vi "Agilent DMM Set Resolution.vi"(7 "Measurement Type":T3, 8 "error in (no error)":errorcluster, 9 "Range":T1, 10 "Resolution":T2, 11 "VISA Resource Name":refnum<visa-resource-name>) -> (0 "error out":errorcluster, 3 "dup VISA Resource Name":refnum<visa-resource-name>)   [LabVIEW 2011]
doc: "This VI for the HP 8753 is used to read the sweep type.\n\n0 LINEAR FREQ\n1 LOG FREQ\n2 LIST FREQ\n3 CW TIME\n4 POWER SWEEP"
uses:
  TypeDefs/Agilent DMM Measurement Type.ctl
  TypeDefs/Agilent DMM Resolution.ctl
  TypeDefs/Agilent DMM Range.ctl
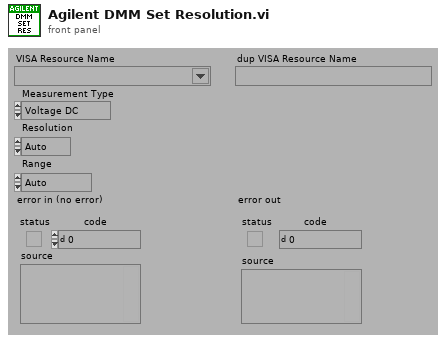
[diagram p1: front panel]
types:
  T1 = typedef "Agilent DMM Range.ctl" = enum16{"Auto", "Min", "Max", "0.01", "0.1", "1", "3", "10", "100", "1,000", "10,000", "100,000", "1,000,000", "10,000,000", "100,000,000"}
  T2 = typedef "Agilent DMM Resolution.ctl" = enum16{"Auto", "Min", "Max", "4 1/2", "5 1/2", "6 1/2"}
  T3 = typedef "Agilent DMM Measurement Type.ctl" = enum16{"Voltage DC", "Voltage DC Ratio", "Voltage AC", "Current DC", "Current AC", "Resistance", "Fresistance", "Frequency", "Period", "Continuity", "Diode"}
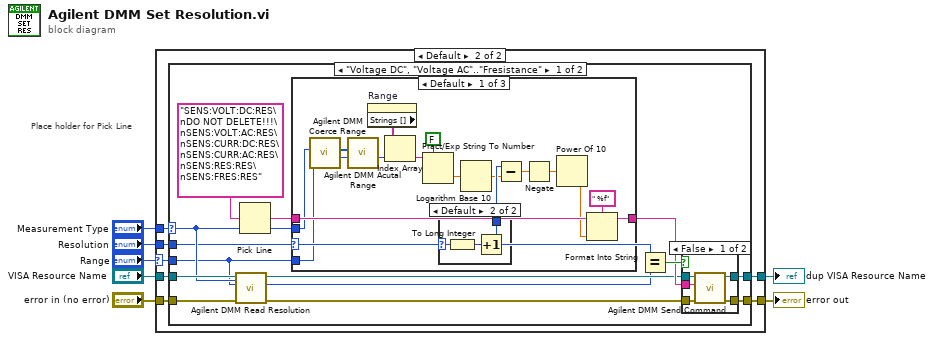
[diagram p0: block diagram]
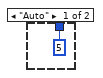
[diagram p4: hidden frame]
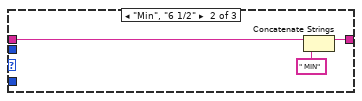
[diagram p5: hidden frame]
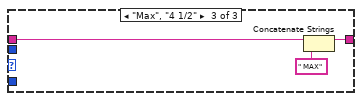
[diagram p6: hidden frame]
diagram:
  # "Place holder for Pick Line"
  n1 = case shown="Default" "Range" {
    selector: "Range" -> [_ w10]
    tunnel: "error in (no error)" -> [w8 w16]
    tunnel: [w8 w15] -> w6
    tunnel: "VISA Resource Name" -> [w9 w14]
    tunnel: [w9 w13] -> w4
    tunnel: "Measurement Type" -> [_ w12]
    tunnel: "Resolution" -> [_ w11]
    frame "Auto" {
      # "The Resolution can only be set\nif the Range is set to something\nbesides Auto."
    }
    frame Default {
      n2 = case shown="\"Voltage DC\", \"Voltage AC\"..\"Fresistance\"" w12 {
        selector: w12 -> [w20 _]
        tunnel: w16 -> [w23 w67]
        tunnel: [w26 w67] -> w15
        tunnel: w14 -> [w24 w66]
        tunnel: [w27 w66] -> w13
        tunnel: w11 -> [w17 _]
        tunnel: w10 -> [w19 _]
        frame "Voltage DC", "Voltage AC".."Fresistance" {
          n3 = call "Agilent DMM Read Resolution.vi"("Measurement Type"=w20, "error in (no error)"=w23, "Range"=w19, "VISA Resource Name"=w24) -> ("error out"=w22:errorcluster, "Resolution"=w18:T2, "dup VISA Resource Name"=w21:refnum<visa-resource-name>)  [unwired: 5 out]
          n4 = Pick Line(multi-line string="SENS:VOLT:DC:RES\nDO NOT DELETE!!!\nSENS:VOLT:AC:RES\nSENS:CURR:DC:RES\nSENS:CURR:AC:RES\nSENS:RES:RES\nSENS:FRES:RES" ("write buffer"), line index=w20) -> (output string=w29:string)  [unwired: 1 out]
          n5 = case shown="Default" w17 {
            selector: w17 -> [w41 _ _]
            tunnel: w29 -> [w54 w61 w64]
            tunnel: [w53 w60 w63] -> w25
            tunnel: w19 -> [w48 _ _]
            tunnel: w20 -> [w47 _ _]
            frame Default {
              n6 = call "Agilent DMM Coerce Range.vi"("Range"=w48, "Measurement Type"=w47) -> ("Coerced Range"=w40:T1, "Available Ranges"=w39:T1[])  [unwired: 8 out]
              n7 = call "Agilent DMM Acutal Range.vi"("Coerced Range"=w40, "Available Ranges"=w39) -> ("Acutal Range"=w38:T1)  [unwired: 9 out]
              n8 = property on="Range" class="Enum (strict)"() -> ("Strings []"=w49:string[])  [unwired: 2 in, 2 out]
              n9 = Index Array(array=w49, index=w38) -> (element=w50:string)
              n10 = Fract/Exp String To Number(use system decimal point (T)=FALSE, string=w50) -> (number=w52:dbl)  [unwired: 3 out]
              n11 = case shown="Default" w41 {
                selector: w41 -> [_ w57]
                tunnel: [5 w59] -> w46
                frame "Auto" {
                }
                frame Default {
                  n12 = To Long Integer(number=w57) -> (32bit integer=w58:i32)
                  n13 = Increment(x=w58) -> (x+1=w59:i32)
                }
              }
              n14 = Logarithm Base 10(1:w52) -> (0:w45:dbl)
              n15 = Subtract(x=w46, y=w45) -> (x-y=w44:dbl)
              n16 = Negate(x=w44) -> (-x=w42:dbl)
              n17 = Power Of 10(x=w42) -> (10^x=w43:dbl)
              n18 = Format Into String(format string=" %f", initial string=w54, w43) -> (resulting string=w53:string)  [unwired: 1 in, 1 out]
            }
            frame "Min", "6 1/2" {
              n19 = Concatenate Strings(w61, " MIN" ("string")) -> (w60:string)
            }
            frame "Max", "4 1/2" {
              n20 = Concatenate Strings(w64, " MAX" ("string")) -> (w63:string)
            }
          }
          n21 = Equal?(x=w17, y=w18) -> (x = y?=w28:bool)
          n22 = case shown="False" w28 {
            tunnel: [w35 w37] -> w27
            tunnel: [w34 w36] -> w26
            tunnel: w25 -> [w33 _]
            tunnel: w21 -> [w32 w37]
            tunnel: w22 -> [w31 w36]
            frame False {
              n23 = call "Agilent DMM Send Command.vi"("error in (no error)"=w31, "Command"=w33, "VISA Resource Name"=w32) -> ("error out"=w34:errorcluster, "dup VISA Resource Name"=w35:refnum<visa-resource-name>)  [unwired: 2 in, 5 out]
            }
            frame True {
            }
          }
        }
        frame Default {
          # "The Resolution can not be set for:\n\nVoltage DC Ratio,\nFrequency,\nPeriod,\nContinuity, or\nDiode."
        }
      }
    }
  }
  "dup VISA Resource Name" <- w4
  "error out" <- w6
